vi "2. Reverse Array.vi"() -> ()   [LabVIEW 2020]
panel:
  out "Array 2":dbl[][](array[numeric])
  in  "Array":dbl[][](array[numeric])=[[1.0, 23.0, 3.0, 4.0, 5.0], [6.0, 7.0, 8.0, 9.0, 10.0], [11.0, 12.0, 13.0, 14.0, 15.0], [16.0, 17.0, 18.0, 19.0, 20.0], [21.0, 22.0, 23.0, 24.0, 25.0]]
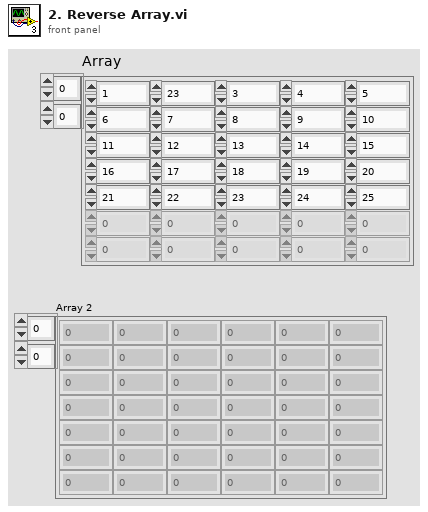
[diagram p1: front panel]
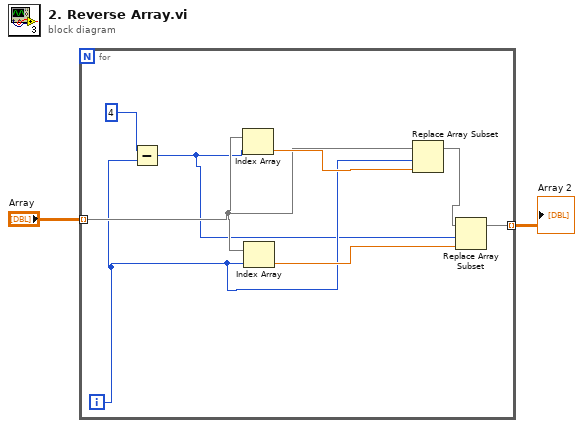
[diagram p0: block diagram]
diagram:
  n1 = for {
    tunnel: "Array" -> [w8] mode=indexing
    tunnel: [w6] -> w1 mode=indexing
    i -> [w4]
    n2 = Subtract(x=4, y=w4) -> (x-y=w3:i32)
    n3 = Index Array(array=w8, index=w3) -> (element=w10:dbl)
    n4 = Index Array(array=w8, index=w4) -> (element=w9:dbl)
    n5 = Replace Array Subset(array=w8, new element=w10, index=w4) -> (w7:dbl[])
    n6 = Replace Array Subset(array=w7, new element=w9, index=w3) -> (w6:dbl[])
  }
  "Array 2" <- w1
